vi "Main.vi"() -> ()   [LabVIEW 2016]
uses:
  StressCalculations/point_data.ctl
  MainFGV/main_FGV_mods.ctl
  MainFGV/main_FGV_data.ctl
  MainFGV/pipe_properties.ctl
  Ovalization/ovalization_data.ctl
  StressDist/StressDist_data.ctl
  StressDist/StressDist_single_data.ctl
  StressDist/Peirce/peirce_data.ctl
  Pressure/pressure_data.ctl
  <vilib>/Analysis/1siggen.llb/Ramp Pattern by Samples.vi
  <vilib>/Analysis/NI_AALBase.lvlib
panel:
  in  "Tab":T1(tab)
  in  "Reload":bool caption="Usar resultados já existentes"
  in  "DiamFuroAndEsp":string caption="Diâmetros do furo e espessuras (opcional)"
  in  "AngAndDiam":string caption="Ângulos e diâmetros em texto (opcional)"
  in  "Pint":dbl[](array[numeric])=[50.0, 50.0, 50.0, 50.0, 50.0] caption="Pressão interna [kgf/cm²]"
  in  "Esp":dbl[](array[numeric])=[11.5, 11.5, 11.6, 11.6, 11.3] caption="Espessura"
  in  "DimCorrect":dbl[](array[numeric])=[1.675, 1.9, 1.93, 1.745, 2.175] caption="Diâmetros corrigidos"
  in  "AngOval":dbl[](array[numeric])=[0.0, 72.0, 144.0, 216.0, 288.0] caption="Ângulos [°]"
  in  "Diams":dbl[](array[numeric])=[608.0, 607.0, 609.57, 607.51, 610.59] caption="Diâmetros duto [mm]"
  in  "e":dbl=11.5 caption="Espessura nominal [mm]"
  in  "Dnom":dbl=609.6 caption="Diâmetro nominal [mm]"
  in  "DirReport":path=path "L:/Documentos/00 SERVIÇOS/Tensão residual/São Sebastião - Osbat/Primeira e segunda seções/Relatorios/Seção 01" caption="Pasta do relatório"
  in  "DirPath":path=path "L:/Documentos/00 SERVIÇOS/Tensão residual/São Sebastião - Osbat/Primeira e segunda seções/Dados/Secao01/FUROS" caption="Caminho dos ensaios"
  out "Error Out":errorcluster
  out "RS_table":string[][](table)
  out "OvalResult":T2
  out "oval_plot":cluster{"X":dbl[], "Y":dbl[]}[](graph) caption="Ovalização"
  # "Dados gerais"
  # "Histórico de pressão"
  # "Ovalização"
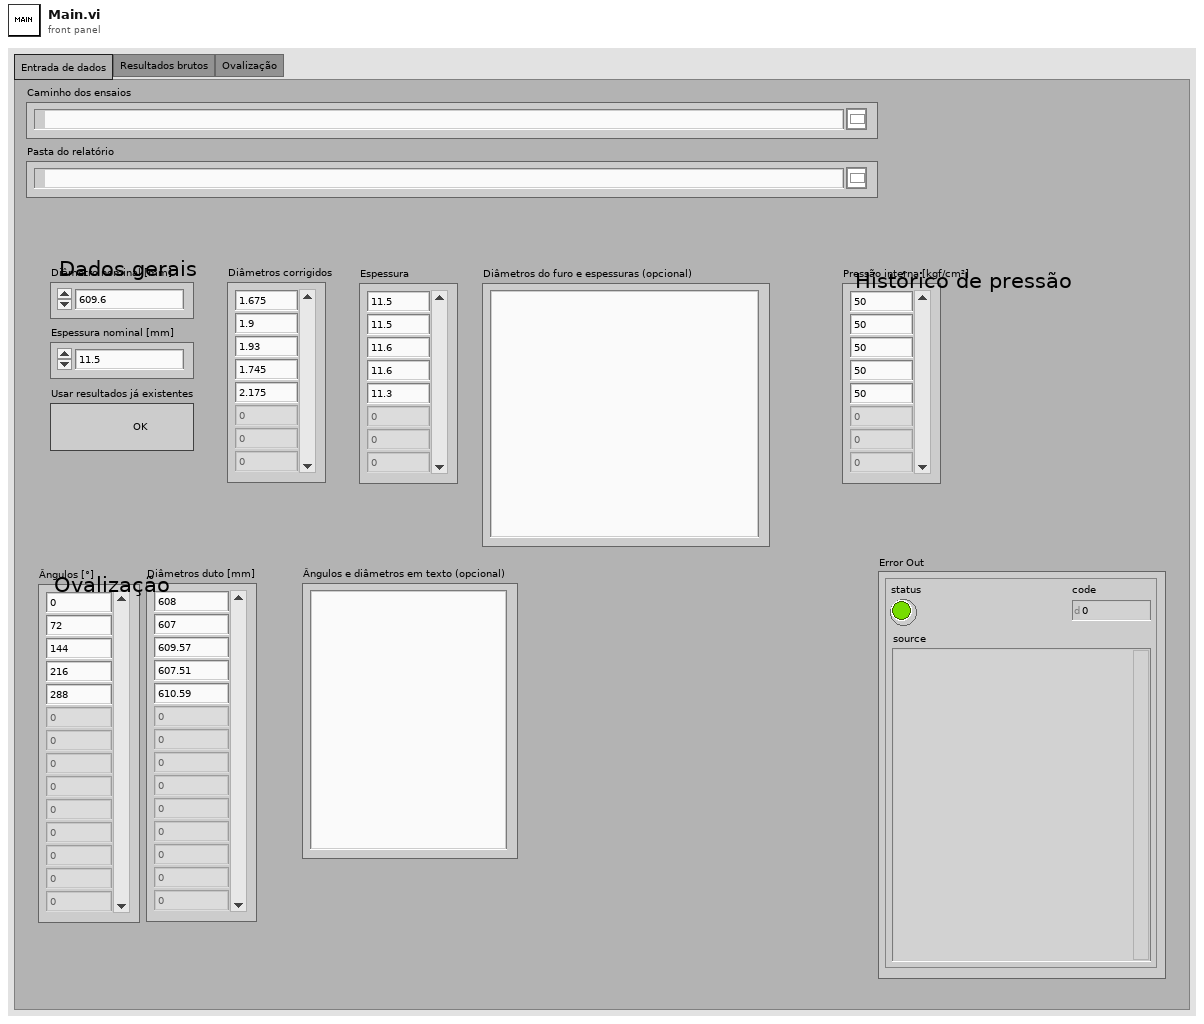
[diagram p1: front panel]
types:
  T1 = enum32{"Entrada de dados", "Resultados brutos", "Ovalização"}
  T2 = cluster{"MD":dbl, "mD":dbl, "Dmed":dbl, "Oval":dbl, "ang":dbl, "X0":dbl, "Y0":dbl}
  T3 = typedef "main_FGV_mods.ctl" = enum16{"Init", "PipeProps", "RSCalc", "Ovalization", "Pressure", "StressDist", "Peirce", "Correct", "End"}
  T4 = typedef "ovalization_data.ctl" = cluster{"AngOval":dbl[], "OvalDiam":dbl[], "Plots":cluster{"Ref":cluster{"X":dbl[], "Y":dbl[]}, "Elipse":cluster{"X":dbl[], "Y":dbl[]}, "Points":cluster{"X":dbl[], "Y":dbl[]}}, "Ampliation":dbl, "Results":cluster{"MD":dbl, "mD":dbl, "Dmed":dbl, "Oval":dbl, "ang":dbl, "X0":dbl, "Y0":dbl}, "fit":dbl[]}
  T5 = typedef "main_FGV_data.ctl" = cluster{"pipe_properties":T6, "DirPath":path, "DirReport":path, "Points":T7[], "ovalization_data":T4, "StressDist_data":T8, "pressure_data":T11, "Reload":bool}
  T6 = typedef "pipe_properties.ctl" = cluster{"out_radius":dbl, "in_radius":dbl, "out_diameter":dbl, "in_diameter":dbl, "thickness":dbl, "inertia":dbl, "area":dbl}
  T7 = typedef "point_data.ctl" = cluster{"LongStress":dbl, "CircStress":dbl, "ShearStress":dbl, "Pressure":dbl, "Angle":dbl, "Thickness":dbl, "HoleDiam":dbl, "EquiStress":dbl, "S1":dbl, "S2":dbl, "Beta":dbl}
  T8 = typedef "StressDist_data.ctl" = cluster{"Long":T9, "Circ":T9, "Shear":T9, "Equivalent":T9}
  T9 = typedef "StressDist_single_data.ctl" = cluster{"Plot":cluster{"Angle":dbl[], "Stress":dbl[]}[], "Fit":dbl[], "ColorMap":dbl[][], "Data":string[][], "peirce_data":T10}
  T10 = typedef "peirce_data.ctl" = cluster{"Plot":cluster{"Array":dbl[], "Array":dbl[]}[], "Index removidos":i32[]}
  T11 = typedef "pressure_data.ctl" = cluster{"Pressure":dbl[], "StressCircOval":dbl[], "StressCirc":dbl[], "StressLong":dbl[], "Plot":cluster{"Angle":dbl[], "Stress":dbl[]}[], "Angle":dbl[]}
  T12 = cluster{"Ref":cluster{"X":dbl[], "Y":dbl[]}, "Elipse":cluster{"X":dbl[], "Y":dbl[]}, "Points":cluster{"X":dbl[], "Y":dbl[]}}
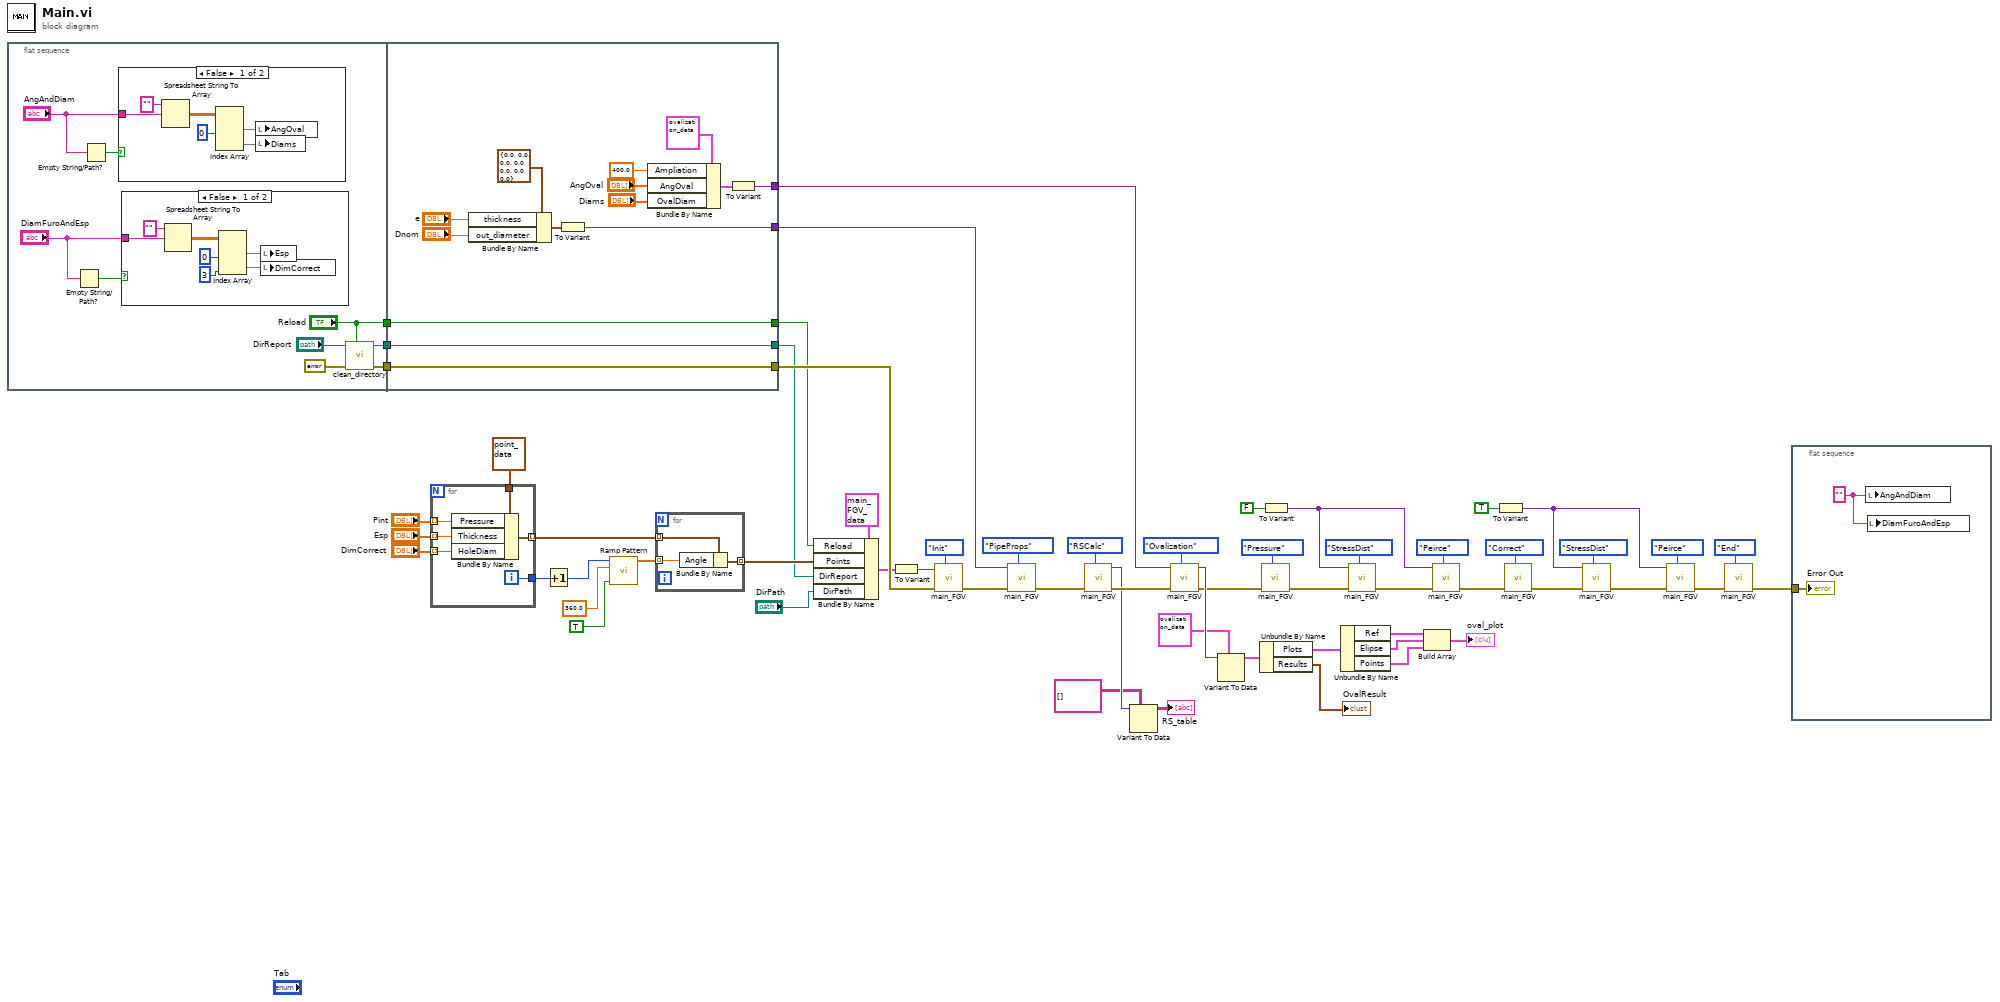
[diagram p0: block diagram]
diagram:
  n1 = flat-sequence {
    tunnel: [w64] -> w43
    tunnel: [w63] -> w42
    tunnel: ["Reload"] -> w37
    tunnel: [w97] -> w61
    tunnel: [w85] -> w39
    tunnel: w43 -> [w85]
    tunnel: w42 -> [w97]
    tunnel: [w87] -> w41
    tunnel: [w86] -> w40
    tunnel: w37 -> [w84]
    tunnel: [w84] -> w36
    frame #0 {
      n2 = Empty String/Path?(string/path="DiamFuroAndEsp") -> (empty?=w69:bool)
      n3 = Empty String/Path?(string/path="AngAndDiam") -> (empty?=w70:bool)
      n4 = case shown="False" w70 {
        tunnel: "AngAndDiam" -> [w83 _]
        frame False {
          n5 = Spreadsheet String To Array(format string="", spreadsheet string=w83) -> (array=w81:dbl[][])  [unwired: 2 in]
          n6 = Index Array(array=w81, index (col) #1=0 ("disabled index (col)")) -> (element #1=w79:dbl[], element #2=w78:dbl[])  [unwired: 3 in]
          n7 = local write "AngOval"(w79) -> ()
          n8 = local write "Diams"(w78) -> ()
        }
        frame True {
        }
      }
      n9 = case shown="False" w69 {
        tunnel: "DiamFuroAndEsp" -> [w77 _]
        frame False {
          n10 = Spreadsheet String To Array(format string="", spreadsheet string=w77) -> (array=w75:dbl[][])  [unwired: 2 in]
          n11 = Index Array(array=w75, index (col) #1=0 ("disabled index (col)"), index (col) #2=3 ("index (col)")) -> (element #1=w73:dbl[], element #2=w72:dbl[])  [unwired: 2 in]
          n12 = local write "Esp"(w73) -> ()
          n13 = local write "DimCorrect"(w72) -> ()
        }
        frame True {
        }
      }
      n14 = call "clean_directory.vi"("Reload"="Reload", "error in"=errorcluster {"status"=FALSE, "code"=0, "source"=""} ("Error In"), "DirReport"="DirReport") -> ("error out"=w63:errorcluster, "DirOut"=w64:path)  [unwired: 7 in]
    }
    frame #1 {
      n15 = Bundle By Name(cluster=T6 {"out_radius"=0.0, "in_radius"=0.0, "out_diameter"=0.0, "in_diameter"=0.0, "thickness"=0.0, "inertia"=0.0, "area"=0.0} ("pipe_properties"), "thickness"="e", "out_diameter"="Dnom") -> (w89:T6)
      n16 = To Variant(anything=w89) -> (Variant=w86:variant)
      n17 = Bundle By Name(cluster=T4 {"AngOval"=[0.0, 60.0, 120.0, 22.5, 45.0, 67.5, 90.0, 112.5, 135.0, 157.5, 180.0], "OvalDiam"=[324.25, 324.6, 324.55, 324.25, 324.55, 324.65, 324.6, 324.65, 324.55, 324.5, 324.4], "Plots"={"Ref"={"X"=[], "Y"=[]}, "Elipse"={"X"=[], "Y"=[]}, "Points"={"X"=[], "Y"=[]}}, "Ampliation"=300.0, "Results"={"MD"=0.0, "mD"=0.0, "Dmed"=0.0, "Oval"=0.0, "ang"=0.0, "X0"=0.0, "Y0"=0.0}, "fit"=[]} ("ovalization_data"), "Ampliation"=400.0, "AngOval"="AngOval", "OvalDiam"="Diams") -> (w95:T4)
      n18 = To Variant(anything=w95) -> (Variant=w87:variant)
    }
  }
  n19 = for {
    tunnel: "Pint" -> [w103] mode=indexing
    tunnel: "Esp" -> [w102] mode=indexing
    tunnel: "DimCorrect" -> [w101] mode=indexing
    tunnel: [w100] -> w57
    tunnel: [w99] -> w55 mode=indexing
    tunnel: T7 {"LongStress"=0.0, "CircStress"=0.0, "ShearStress"=0.0, "Pressure"=0.0, "Angle"=0.0, "Thickness"=0.0, "HoleDiam"=0.0, "EquiStress"=0.0, "S1"=0.0, "S2"=0.0, "Beta"=0.0} ("point_data") -> [w98]
    i -> [w100]
    n20 = Bundle By Name(cluster=w98, "Pressure"=w103, "Thickness"=w102, "HoleDiam"=w101) -> (w99:T7)
  }
  n21 = Increment(x=w57) -> (x+1=w52:i32)
  n22 = call-poly <vilib>:"Ramp Pattern.vi"("exclude end?"=TRUE, "end"=360.0, "samples"=w52) -> ("Ramp Pattern"=w54:dbl[])  [unwired: 7 in, 1 out]
  n23 = for {
    tunnel: w55 -> [w106] mode=indexing
    tunnel: w54 -> [w105] mode=indexing
    tunnel: [w104] -> w47 mode=indexing
    n24 = Bundle By Name(cluster=w106, "Angle"=w105) -> (w104:T7)
  }
  n25 = Bundle By Name(cluster=T5 {"pipe_properties"={"out_radius"=0.0, "in_radius"=0.0, "out_diameter"=0.0, "in_diameter"=0.0, "thickness"=0.0, "inertia"=0.0, "area"=0.0}, "DirPath"=path "L:/Documentos/00 SERVIÇOS/Tensão residual/Olapa 10-2017/Dados/Primeira Seção/Furos", "DirReport"=path "L:/Documentos/00 SERVIÇOS/Tensão residual/Olapa 10-2017/RelatóriosOlapa/Teste", "Points"=[], "ovalization_data"={"AngOval"=[0.0, 60.0, 120.0, 22.5, 45.0, 67.5, 90.0, 112.5, 135.0, 157.5, 180.0], "OvalDiam"=[324.25, 324.6, 324.55, 324.25, 324.55, 324.65, 324.6, 324.65, 324.55, 324.5, 324.4], "Plots"={"Ref"={"X"=[], "Y"=[]}, "Elipse"={"X"=[], "Y"=[]}, "Points"={"X"=[], "Y"=[]}}, "Ampliation"=100.0, "Results"={"MD"=0.0, "mD"=0.0, "Dmed"=0.0, "Oval"=0.0, "ang"=0.0, "X0"=0.0, "Y0"=0.0}, "fit"=[]}, "StressDist_data"={"Long"={"Plot"=[], "Fit"=[], "ColorMap"=[], "Data"=[], "peirce_data"={"Plot"=[], "Index removidos"=[]}}, "Circ"={"Plot"=[], "Fit"=[], "ColorMap"=[], "Data"=[], "peirce_data"={"Plot"=[], "Index removidos"=[]}}, "Shear"={"Plot"=[], "Fit"=[], "ColorMap"=[], "Data"=[], "peirce_data"={"Plot"=[], "Index removidos"=[]}}, "Equivalent"={"Plot"=[], "Fit"=[], "ColorMap"=[], "Data"=[], "peirce_data"={"Plot"=[], "Index removidos"=[]}}}, "pressure_data"={"Pressure"=[], "StressCircOval"=[], "StressCirc"=[], "StressLong"=[], "Plot"=[], "Angle"=[]}, "Reload"=FALSE} ("main_FGV_data"), "Reload"=w36, "Points"=w47, "DirReport"=w39, "DirPath"="DirPath") -> (w46:T5)
  n26 = To Variant(anything=w46) -> (Variant=w50:variant)
  n27 = call "main_FGV.vi"("main_FGV_mods"=main_FGV_mods."Init", "Error In"=w61, "ParamIn"=w50) -> ("Error Out"=w49:errorcluster)  [unwired: 7 in, 1 out]
  n28 = call "main_FGV.vi"("main_FGV_mods"=main_FGV_mods."PipeProps", "Error In"=w49, "ParamIn"=w40) -> ("Error Out"=w33:errorcluster)  [unwired: 7 in, 1 out]
  n29 = call "main_FGV.vi"("main_FGV_mods"=main_FGV_mods."RSCalc", "Error In"=w33) -> ("Error Out"=w32:errorcluster, "ParamOut"=w31:variant)  [unwired: 8 in]
  n30 = Variant To Data(type=string[][] [] ("Table"), Variant=w31) -> (data=→"RS_table":string[][])  [unwired: 1 in, 1 out]
  n31 = call "main_FGV.vi"("main_FGV_mods"=main_FGV_mods."Ovalization", "Error In"=w32, "ParamIn"=w41) -> ("Error Out"=w13:errorcluster, "ParamOut"=w27:variant)  [unwired: 7 in]
  n32 = Variant To Data(type=T4 {"AngOval"=[0.0, 60.0, 120.0, 22.5, 45.0, 67.5, 90.0, 112.5, 135.0, 157.5, 180.0], "OvalDiam"=[324.25, 324.6, 324.55, 324.25, 324.55, 324.65, 324.6, 324.65, 324.55, 324.5, 324.4], "Plots"={"Ref"={"X"=[], "Y"=[]}, "Elipse"={"X"=[], "Y"=[]}, "Points"={"X"=[], "Y"=[]}}, "Ampliation"=100.0, "Results"={"MD"=0.0, "mD"=0.0, "Dmed"=0.0, "Oval"=0.0, "ang"=0.0, "X0"=0.0, "Y0"=0.0}, "fit"=[]} ("ovalization_data"), Variant=w27) -> (data=w20:T4)  [unwired: 1 in, 1 out]
  n33 = Unbundle By Name(w20) -> ("Plots"=w25:T12, "Results"=→"OvalResult":T2)
  n34 = call "main_FGV.vi"("main_FGV_mods"=main_FGV_mods."Pressure", "Error In"=w13) -> ("Error Out"=w12:errorcluster)  [unwired: 8 in, 1 out]
  n35 = To Variant(anything=FALSE ("exclude end?")) -> (Variant=w10:variant)
  n36 = Unbundle By Name(w25) -> ("Ref"=w24:cluster{"X":dbl[], "Y":dbl[]}, "Elipse"=w21:cluster{"X":dbl[], "Y":dbl[]}, "Points"=w22:cluster{"X":dbl[], "Y":dbl[]})
  n37 = call "main_FGV.vi"("main_FGV_mods"=main_FGV_mods."StressDist", "Error In"=w12, "ParamIn"=w10) -> ("Error Out"=w15:errorcluster)  [unwired: 7 in, 1 out]
  n38 = Build Array(w24, w21, w22) -> (→"oval_plot":cluster{"X":dbl[], "Y":dbl[]}[])
  n39 = call "main_FGV.vi"("main_FGV_mods"=main_FGV_mods."Peirce", "Error In"=w15, "ParamIn"=w10) -> ("Error Out"=w8:errorcluster)  [unwired: 7 in, 1 out]
  n40 = To Variant(anything=TRUE ("exclude end?")) -> (Variant=w7:variant)
  n41 = call "main_FGV.vi"("main_FGV_mods"=main_FGV_mods."Correct", "Error In"=w8) -> ("Error Out"=w2:errorcluster)  [unwired: 8 in, 1 out]
  n42 = call "main_FGV.vi"("main_FGV_mods"=main_FGV_mods."StressDist", "Error In"=w2, "ParamIn"=w7) -> ("Error Out"=w5:errorcluster)  [unwired: 7 in, 1 out]
  n43 = call "main_FGV.vi"("main_FGV_mods"=main_FGV_mods."Peirce", "Error In"=w5, "ParamIn"=w7) -> ("Error Out"=w1:errorcluster)  [unwired: 7 in, 1 out]
  n44 = call "main_FGV.vi"("main_FGV_mods"=main_FGV_mods."End", "Error In"=w1) -> ("Error Out"=w38:errorcluster)  [unwired: 8 in, 1 out]
  n45 = flat-sequence {
    tunnel: w38 -> [w108]
    frame #0 {
      w107 = "" ("AngAndDiam")
      n46 = local write "AngAndDiam"(w107) -> ()
      n47 = local write "DiamFuroAndEsp"(w107) -> ()
      "Error Out" <- w108
    }
  }
